vi "IAmGLF-New.vi"(8 "error in (no error)":errorcluster, 10 "Data":variant, 11 "IAmGLF in":refnum<class "IAmGLF.lvclass">) -> (0 "error out":errorcluster, 3 "IAmGLF out":refnum<class "IAmGLF.lvclass">)   [LabVIEW 2024, in "GLF.lvlib" / "IAmGLF.lvclass"]
doc: "<B>Summary</B>\nCreates a new instance of the given GLF object. For internal use only."
uses:
  IAmGLF.lvclass
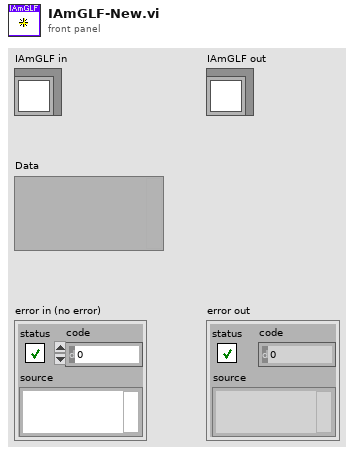
[diagram p1: front panel]
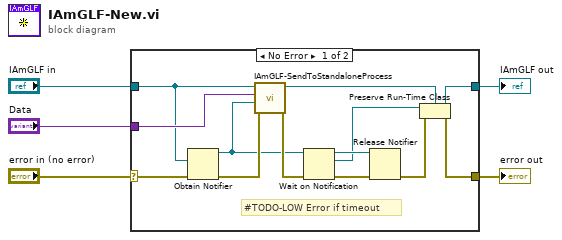
[diagram p0: block diagram]
diagram:
  n1 = case shown="No Error" "error in (no error)" {
    selector: "error in (no error)" -> [w16 w20]
    tunnel: [w12 w20] -> w4
    tunnel: [w14 w19] -> w2
    tunnel: "IAmGLF in" -> [w7 w19]
    tunnel: "Data" -> [w9 _]
    frame No Error {
      # "#TODO-LOW Error if timeout"
      n2 = Obtain Notifier(notification data type=w7, error in (no error)=w16) -> (notifier out=w6:refnum<notifier>, error out=w11:errorcluster)  [unwired: 2 in, 1 out]
      n3 = call-dynamic "IAmGLF-SendToStandaloneProcess.vi"("error in (no error)"=w11, "Class Return Notifier"=w6, "Data"=w9, "IAmGLF in"=w7) -> ("error out"=w10:errorcluster, "IAmGLF out"=w8:refnum<class "IAmGLF.lvclass">)  [unwired: 6 in]
      n4 = Wait on Notification(notifier=w6, error in (no error)=w10) -> (notifier out=w18:refnum<notifier>, notification=w15:refnum<class "IAmGLF.lvclass">, error out=w17:errorcluster)  [unwired: 2 in, 1 out]
      n5 = Release Notifier(notifier=w18, error in (no error)=w17) -> (error out=w13:errorcluster)  [unwired: 1 in, 2 out]
      n6 = Preserve Run-Time Class(object in=w15, error in=w13, 2:w8) -> (object out=w14:refnum<class "IAmGLF.lvclass">, error out=w12:errorcluster)
    }
    frame Error {
    }
  }
  "error out" <- w4
  "IAmGLF out" <- w2
